vi "E8267D GetErrors.vi"(0 "VISA Rsrc":refnum<visa-resource-name>="GPIB0::12::INSTR", 11 "error in (no error)":errorcluster) -> (4 "VISA Rsrc Out":refnum<visa-resource-name>="GPIB0::12::INSTR", 6 "Err String":string, 8 "Errors":bool, 15 "error out":errorcluster)   [LabVIEW 2019]
doc: "Ce VI écrit les paramètres de la zone de contrôle spécifiée dans le contrôlleur"
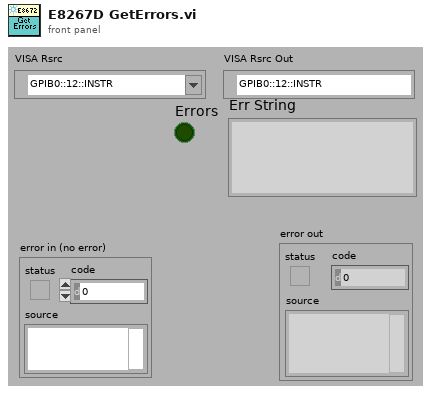
[diagram p1: front panel]
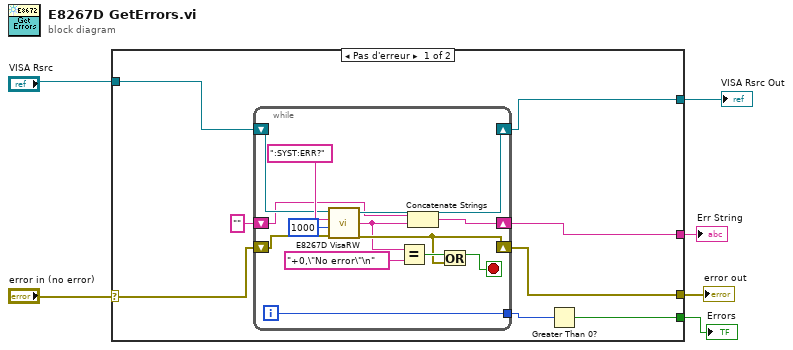
[diagram p0: block diagram]
diagram:
  n1 = case shown="Pas d'erreur" "error in (no error)" {
    selector: "error in (no error)" -> [w12 w29]
    tunnel: "VISA Rsrc" -> [w13 w28]
    tunnel: [w11 w29] -> w5
    tunnel: [w14 w28] -> w3
    tunnel: [w9 _] -> w2
    tunnel: [w7 _] -> w1
    frame No Error {
      n2 = while {
        shift-right: [w27] -> w14
        shift-left: w13 -> [w25]
        shift-right: [w19] -> w11
        shift-left: w12 -> [w24]
        shift-right: [w17] -> w9
        shift-left: "" -> [w16]
        tunnel: [w15] -> w8
        i -> [w15]
        stop <- w20 stop-if-true
        n3 = call <userlib>:"E8267D VisaRW.vi"("error in (no error)"=w24, "Nbcaract"=u32 1000, "ChaineCom"=":SYST:ERR?" ("true string"), "VISA Rsrc"=w25) -> ("error out"=w19:errorcluster, "ChaineRep"=w18:string, "VISA Rsrc Out"=w27:refnum<visa-resource-name>)  [unwired: 3 in, 1 out]
        n4 = Equal?(x=w18, y="+0,\"No error\"\n" ("true string")) -> (x = y?=w21:bool)
        n5 = Concatenate Strings(w16, w18) -> (w17:string)
        n6 = Or(x=w21, y=w19) -> (x .or. y?=w20:bool)
      }
      n7 = Greater Than 0?(x=w8) -> (x > 0?=w7:bool)
    }
    frame Error {
    }
  }
  "error out" <- w5
  "VISA Rsrc Out" <- w3
  "Err String" <- w2
  "Errors" <- w1
